vi "txrx.vi"() -> ()   [LabVIEW 2014]
doc: "TxRx\nRegistra un segnale su CB68 con trigger (CB10)"
uses:
  <vilib>/DAQmx/read.llb/DAQmx Read (Analog Wfm 1Chan NSamp).vi
  <vilib>/DAQmx/create/channels.llb/DAQmx Create Channel (AI-Voltage-Basic).vi
  <vilib>/DAQmx/configure/timing.llb/DAQmx Timing (Sample Clock).vi
  <vilib>/DAQmx/configure/trigger.llb/DAQmx Reference Trigger (Digital Edge).vi
  <vilib>/DAQmx/miscellaneous.llb/DAQmx Fill In Error Info.vi
panel:
  in  "stop":bool
  out "delta T (ms)":dbl=0.11199999999999968 format="%_4f"
  in  "durata (ms)":dbl=1.2
  out "Waveform Graph":waveform(dbl)(graph)={"t0"=timestamp(3478231731.968892 s since 1904-01-01), "dt"=3.999999999999989e-06, "Y"=array[2500 elements], "attributes"=variant("NI_ChannelName"=variant(string "Dev1/ai0"), "NI_UnitDescription"=variant(string "Volts"))}
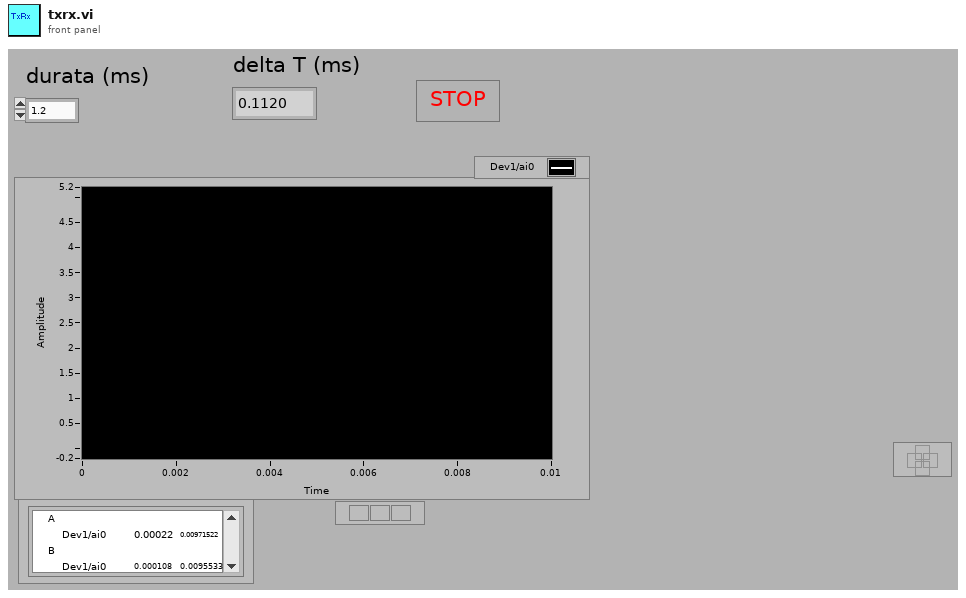
[diagram p1: front panel]
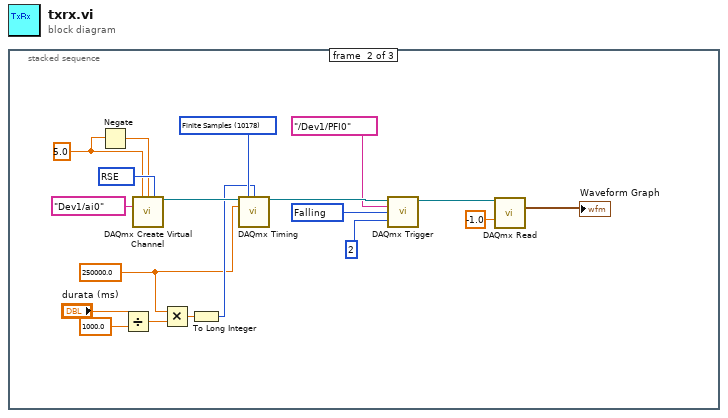
[diagram p0: block diagram]
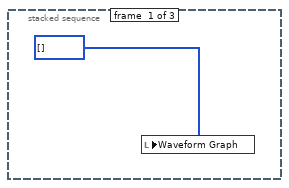
[diagram p2: hidden frame]
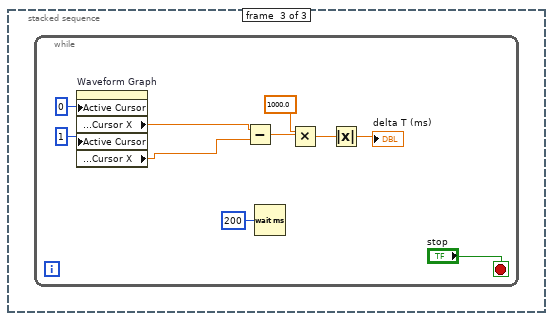
[diagram p3: hidden frame]
diagram:
  n1 = stacked-sequence {
    frame #0 {
      n2 = local write "Waveform Graph"(i32[] []) -> ()
    }
    frame #1 {
      w2 = 5.0 ("maximum value")
      w11 = 10178 items=["Finite Samples"=10178, "Continuous Samples"=10123, "Hardware Timed Single Point"=12522] ("sample mode")
      w13 = 10171 items=["Rising"=10280, "Falling"=10171] ("edge")
      w17 = 10083 items=["default"=-1, "RSE"=10083, "NRSE"=10078, "Differential"=10106, "Pseudodifferential"=12529] ("input terminal configuration")
      w3 = 250000.0 ("rate")
      n3 = Negate(x=w2) -> (-x=w10:dbl)
      n4 = Divide(x="durata (ms)", y=1000.0) -> (x/y=w4:dbl)
      n5 = call-poly <vilib>:"DAQmx Create Virtual Channel.vi"("maximum value"=w2, "minimum value"=w10, "input terminal configuration"=w17, "physical channels"=tag "Dev1/ai0") -> ("task out"=w19:refnum<k21>)  [unwired: 5 in, 6 out]
      n6 = Multiply(x=w3, y=w4) -> (x*y=w8:dbl)
      n7 = To Long Integer(number=w8) -> (32bit integer=w6:i32)
      n8 = call-poly <vilib>:"DAQmx Timing.vi"("task/channels in"=w19, "sample mode"=w11, "samples per channel"=w6, "rate"=w3) -> ("task out"=w16:refnum<k21>)  [unwired: 3 in, 8 out]
      n9 = call-poly <vilib>:"DAQmx Trigger.vi"("task/channels in"=w16, "source"=tag "/Dev1/PFI0", "edge"=w13, "pretrigger samples per channel"=u32 2) -> ("task out"=w15:refnum<k21>)  [unwired: 1 in, 10 out]
      n10 = call-poly <vilib>:"DAQmx Read.vi"("task/channels in"=w15, "timeout"=-1.0) -> ("data"=→"Waveform Graph":waveform(dbl))  [unwired: 2 in, 11 out]
    }
    frame #2 {
      n11 = while {
        stop <- "stop" stop-if-true
        n12 = property on="Waveform Graph" class="WFGraph (strict)"("Active Cursor"=0 ("Cursor.Cursor Index"), "Active Cursor"=1 ("Cursor.Cursor Index")) -> ("Cursor.Cursor Position:Cursor X"=w28:dbl, "Cursor.Cursor Position:Cursor X"=w27:dbl)  [unwired: 2 in, 2 out]
        n13 = Subtract(x=w28, y=w27) -> (x-y=w26:dbl)
        n14 = Wait (ms)(milliseconds to wait=u32 200) -> ()  [unwired: 1 out]
        n15 = Multiply(x=1000.0, y=w26) -> (x*y=w22:dbl)
        n16 = Absolute Value(x=w22) -> (abs(x)=→"delta T (ms)":dbl)
      }
    }
  }
